vi "GetEvents.vi"(8 "error in (no error)":errorcluster, 11 "CameraTesting in":refnum<class "CameraTesting.lvclass">) -> (0 "error out":errorcluster, 3 "CameraTesting out":refnum<class "CameraTesting.lvclass">)   [LabVIEW 2020, in "CameraTesting.lvlib" / "CameraTesting.lvclass"]
uses:
  CameraTesting.lvclass
  <vilib>/ActorFramework/Message Enqueuer/Message Priority.ctl
  CameraTesting.lvclass/CameraTesting.ctl
  ICameraTestingUI/ICameraTestingUI Messages/CamTestGetEvntsResponse Msg/CamTestGetEvntsResponse Msg.lvclass/CamTestGetEvntsResponse Msg.ctl
  <vilib>/ActorFramework/Message Enqueuer/Message Enqueuer.lvclass/Message Enqueuer.ctl
  <vilib>/ActorFramework/Message Enqueuer/Enqueue.vi
  ICameraTestingUI/ICameraTestingUI Messages/CamTestGetEvntsResponse Msg/CamTestGetEvntsResponse Msg.lvclass
  C:/Program Files (x86)/National Instruments/LabVIEW 2020/vi.lib/ActorFramework/Message/Message.lvclass
  <vilib>/ActorFramework/Message Priority Queue/Priority Enqueue.vi
  <vilib>/ActorFramework/Message Enqueuer/Message Enqueuer.lvclass
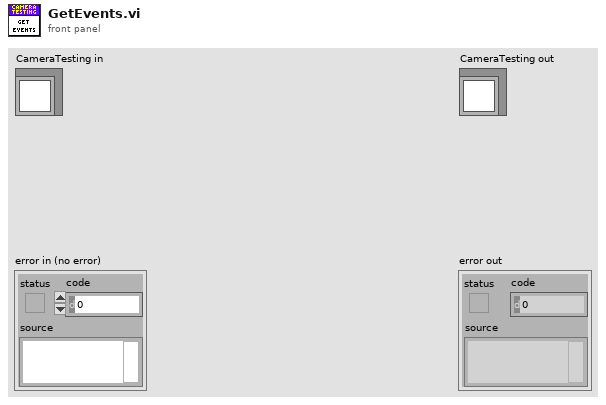
[diagram p1: front panel]
types:
  T1 = typedef "Actor Framework.lvlib/Message Enqueuer.lvclass/Message Priority.ctl" = enum16{"Low", "Normal", "High"}
  T2 = typedef "ICameraTesting.lvlib/ICameraTesting.lvclass/Events.ctl" = cluster{"NewSnapData":refnum<user-event>, "FrameRateValReceived":T3, "ImgTypeValReceived":T4, "ResolutionValReceived":T5, "VideoOptInfoUpdated":T6, "StatusUpdated":T7, "VideoBufferUpdate":T8}
  T3 = typedef "ICameraTesting.lvlib/ICameraTesting.lvclass/FrameRateValReceived.ctl" = refnum<user-event>
  T4 = typedef "ICameraTesting.lvlib/ICameraTesting.lvclass/ImgTypeValReceived.ctl" = refnum<user-event>
  T5 = typedef "ICameraTesting.lvlib/ICameraTesting.lvclass/ResolutionValReceived.ctl" = refnum<user-event>
  T6 = typedef "ICameraTesting.lvlib/ICameraTesting.lvclass/VideoOptCodesUpdated.ctl" = refnum<user-event>
  T7 = typedef "ICameraTesting.lvlib/ICameraTesting.lvclass/StatusUpdated.ctl" = refnum<user-event>
  T8 = typedef "ICameraTesting.lvlib/ICameraTesting.lvclass/VideoBufferUpdate.ctl" = refnum<user-event>
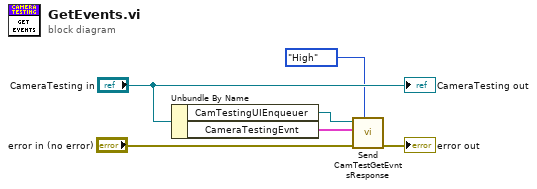
[diagram p0: block diagram]
diagram:
  n1 = Unbundle By Name("CameraTesting in") -> ("CamTestingUIEnqueuer"=w5:refnum<class "Message Enqueuer.lvclass">, "CameraTestingEvnt"=w4:T2)
  n2 = call "Send CamTestGetEvntsResponse.vi"("Message Priority (Normal)"=Message_Priority."High", "error in (no error)"="error in (no error)", "CameraTestingEvnt"=w4, "Message Enqueuer"=w5) -> ("error out"=→"error out":errorcluster)  [unwired: 6 in, 1 out]
  "CameraTesting out" <- "CameraTesting in"
